vi "Edit Config.vi"(8 "error in (no error)":errorcluster, 11 "Scaling in":refnum<class "Scaling.lvclass">) -> (0 "error out":errorcluster, 3 "Scaling out":refnum<class "Scaling.lvclass">)   [LabVIEW 2018, in "Scaling.lvclass"]
doc: "Scaling.lvclass:Edit Config.vi\n\nThis VI is the template for the Edit Config VI for the Scaling class.\n\nInstrument Communication Module Version 1.0\nSeptember, 2017 Original Code Consulting David Thomson\n www.originalcode.com"
uses:
  Scaling.lvclass
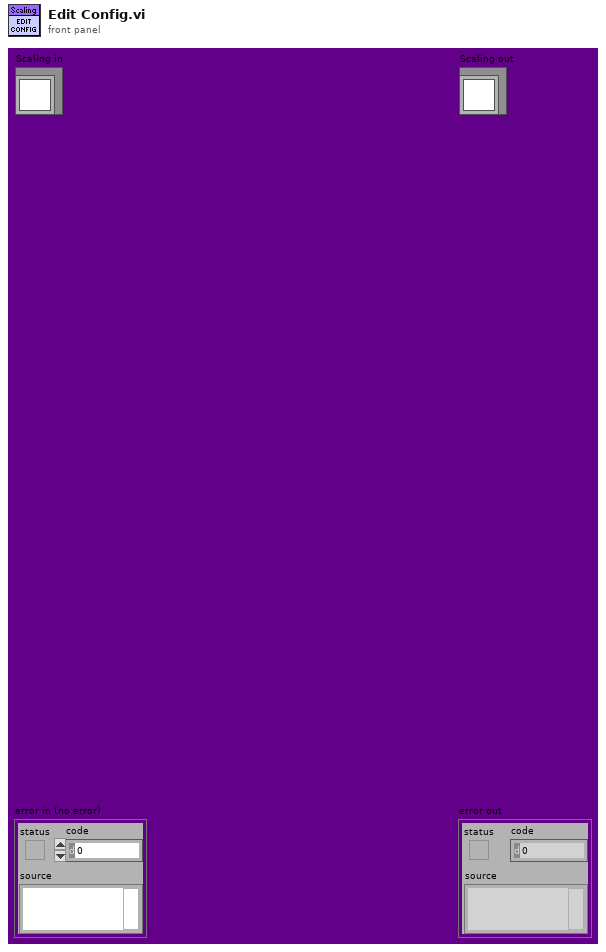
[diagram p1: front panel]
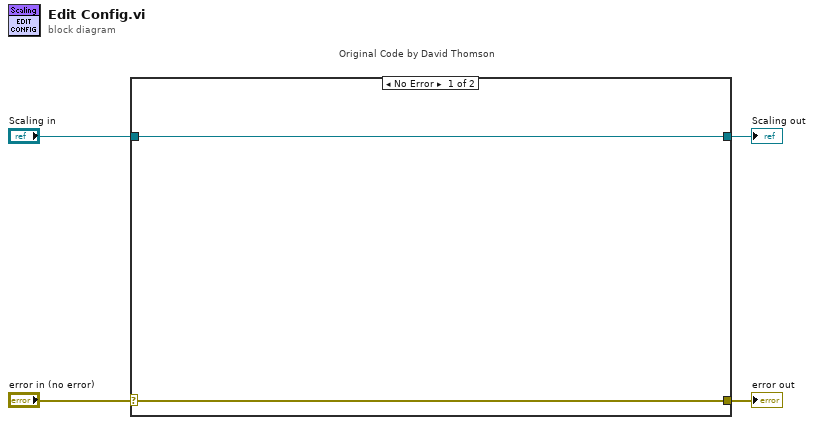
[diagram p0: block diagram]
diagram:
  n1 = case "Original Code by David Thomson" shown="No Error" "error in (no error)" {
    selector: "error in (no error)" -> [w5 w8]
    tunnel: [w5 w8] -> w3
    tunnel: [w6 w7] -> w1
    tunnel: "Scaling in" -> [w6 w7]
    frame No Error {
    }
    frame Error {
    }
  }
  "error out" <- w3
  "Scaling out" <- w1
